vi "Serial fit Lc and K.vi"(0 "Extension (nm)":dbl[](array[numeric]), 2 "Force (pN)":dbl[](array[numeric]), 3 "initial parameters for WLC (Lp,Lc)":dbl[](array[numeric])=[45.0, 1800.0]) -> (1 "Cut-Extenison (nm)":dbl[](array[numeric]), 4 "Cut-Force (pN)":dbl[](array[numeric]), 6 "best fit parameters for eWLC (Lp,Lc,K)":dbl[](array[numeric]), 7 "best fit parameters for WLC":dbl[](array[numeric]), 8 "best nonlinear fit extension for eWLC":dbl[](array[numeric]))   [LabVIEW 2014]
uses:
  <vilib>/gmath/NumericalOptimization/Nonlinear Curve Fit LM formula string.vi
  <vilib>/gmath/NI_Gmath.lvlib
panel:
  out "error out 2":errorcluster
  out "error out":errorcluster
  out "Lp (nm)":dbl
  out "Model to fit":string
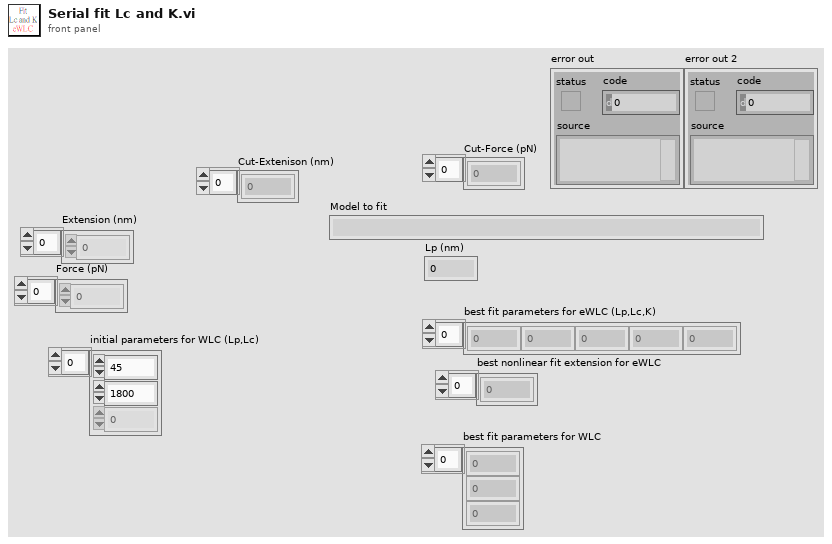
[diagram p1: front panel]
types:
  T1 = cluster{"model":string, "Parameters":string[], "x":string}
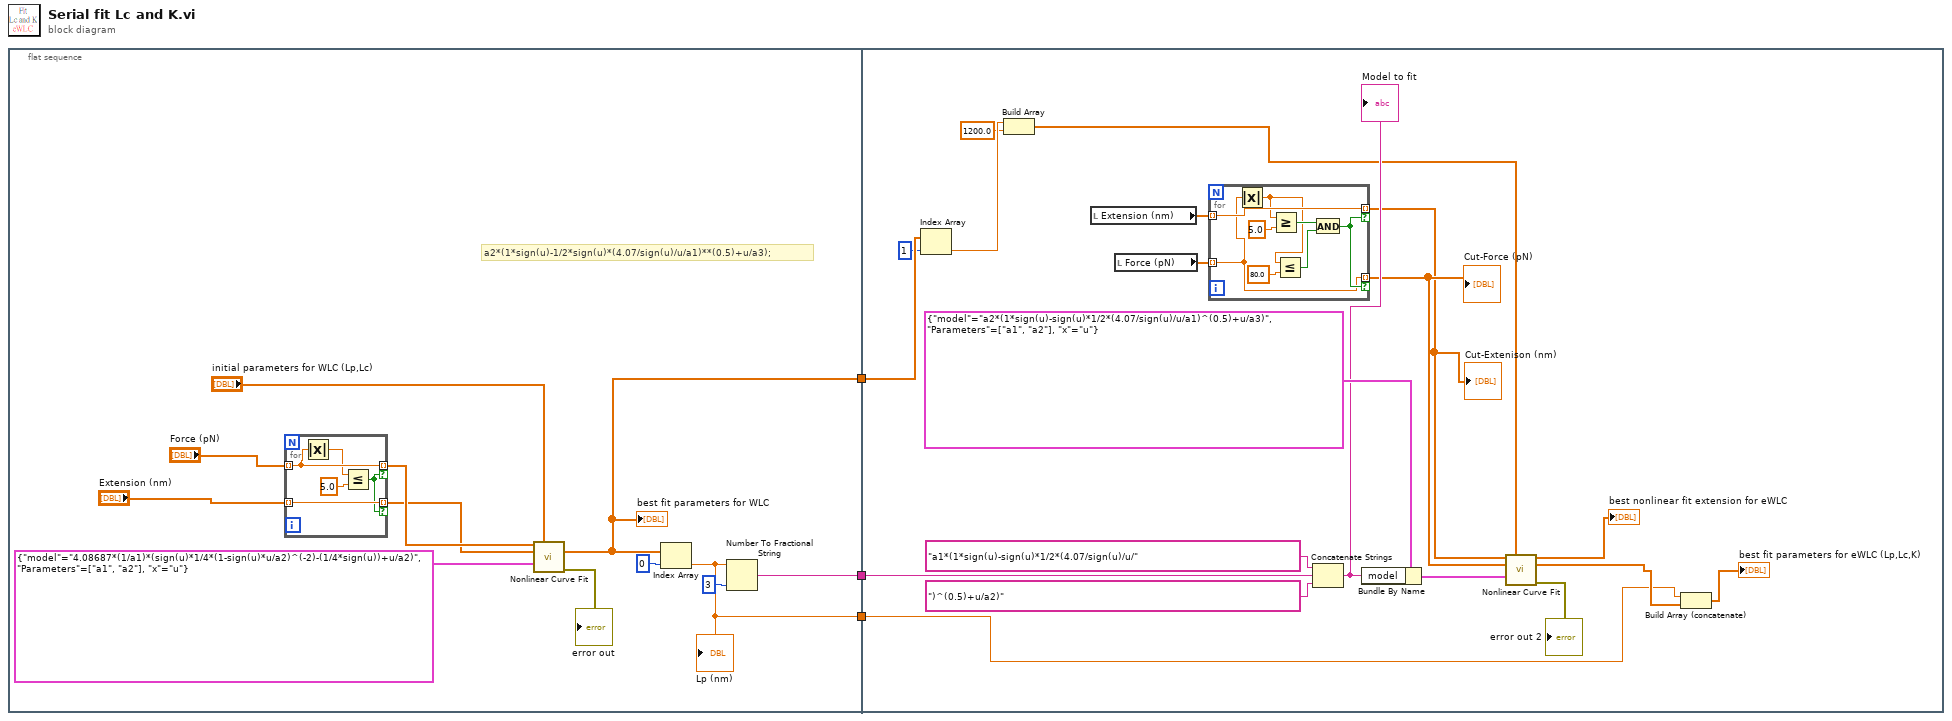
[diagram p0: block diagram]
diagram:
  n1 = flat-sequence {
    tunnel: [w12] -> w3
    tunnel: [w7] -> w2
    tunnel: [w5] -> w1
    tunnel: w3 -> [w38]
    tunnel: w2 -> [w29]
    tunnel: w1 -> [w26]
    frame #0 {
      # "a2*(1*sign(u)-1/2*sign(u)*(4.07/sign(u)/u/a1)**(0.5)+u/a3);"
      n2 = for {
        tunnel: "Force (pN)" -> [w17] mode=indexing
        tunnel: [w17] -> w9 mode=indexing if=w18
        tunnel: "Extension (nm)" -> [w19] mode=indexing
        tunnel: [w19] -> w8 mode=indexing if=w18
        n3 = Absolute Value(x=w17) -> (abs(x)=w16:dbl)
        n4 = Less Or Equal?(x=w16, y=5.0) -> (x <= y?=w18:bool)
      }
      n5 = call-poly <vilib>:"Nonlinear Curve Fit.vi"("Y"=w9, "initial parameters"="initial parameters for WLC (Lp,Lc)", "X"=w8, "model description"=T1 {"model"="4.08687*(1/a1)*(sign(u)*1/4*(1-sign(u)*u/a2)^(-2)-(1/4*sign(u))+u/a2)", "Parameters"=["a1", "a2"], "x"="u"}) -> ("best fit parameters"=w5:dbl[], "error out"=→"error out":errorcluster)  [unwired: 3 in, 7 out]
      "best fit parameters for WLC" <- w5
      n6 = Index Array(array=w5, index=0) -> (element=w7:dbl)
      "Lp (nm)" <- w7
      n7 = Number To Fractional String(number=w7, precision (6)=i16 3) -> (F-format string=w12:string)  [unwired: 2 in]
    }
    frame #1 {
      n8 = Index Array(array=w26, index=1) -> (element=w24:dbl)
      n9 = Build Array(w24, 1200.0 ("element")) -> (w22:dbl[])
      n10 = local read "Extension (nm)"() -> (w32:dbl[])
      n11 = local read "Force (pN)"() -> (w33:dbl[])
      n12 = for {
        tunnel: w33 -> [w42] mode=indexing
        tunnel: [w42] -> w31 mode=indexing if=w43
        tunnel: w32 -> [w47] mode=indexing
        tunnel: [w47] -> w27 mode=indexing if=w43
        n13 = Absolute Value(x=w42) -> (abs(x)=w41:dbl)
        n14 = Greater Or Equal?(x=w41, y=5.0) -> (x >= y?=w45:bool)
        n15 = Less Or Equal?(x=w41, y=80.0) -> (x <= y?=w44:bool)
        n16 = And(x=w45, y=w44) -> (x .and. y?=w43:bool)
      }
      "Cut-Force (pN)" <- w31
      "Cut-Extenison (nm)" <- w27
      n17 = Concatenate Strings("a1*(1*sign(u)-sign(u)*1/2*(4.07/sign(u)/u/" ("model"), w38, ")^(0.5)+u/a2)" ("model")) -> (w36:string)
      "Model to fit" <- w36
      n18 = Bundle By Name(cluster=T1 {"model"="a2*(1*sign(u)-sign(u)*1/2*(4.07/sign(u)/u/a1)^(0.5)+u/a3)", "Parameters"=["a1", "a2"], "x"="u"} ("model description"), "model"=w36) -> (w35:T1)
      n19 = call-poly <vilib>:"Nonlinear Curve Fit.vi"("Y"=w27, "initial parameters"=w22, "X"=w31, "model description"=w35) -> ("best nonlinear fit"=→"best nonlinear fit extension for eWLC":dbl[], "best fit parameters"=w30:dbl[], "error out"=→"error out 2":errorcluster)  [unwired: 3 in, 6 out]
      n20 = Build Array (concatenate)(w29, w30) -> (→"best fit parameters for eWLC (Lp,Lc,K)":dbl[])
    }
  }
